vi "Leng Conv.vi"(8 "Unit":bool, 11 "Winding Length":dbl) -> (3 "String":string)   [LabVIEW 2014, in "Programing Logic.lvclass"]
uses:
  Programming Logic/Programing Logic.lvclass
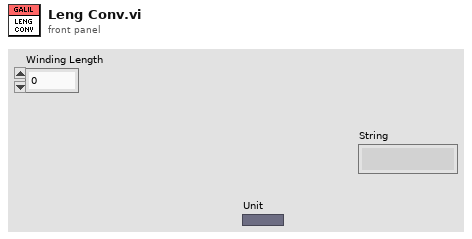
[diagram p1: front panel]
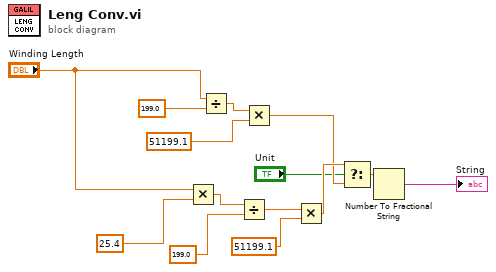
[diagram p0: block diagram]
diagram:
  n1 = Multiply(x="Winding Length", y=25.4) -> (x*y=w6:dbl)
  n2 = Divide(x="Winding Length", y=199.0) -> (x/y=w3:dbl)
  n3 = Divide(x=w6, y=199.0) -> (x/y=w10:dbl)
  n4 = Multiply(x=w3, y=51199.1) -> (x*y=w13:dbl)
  n5 = Multiply(x=w10, y=51199.1) -> (x*y=w14:dbl)
  n6 = Select(t=w14, s="Unit", f=w13) -> (s? t:f=w8:dbl)
  n7 = Number To Fractional String(number=w8) -> (F-format string=→"String":string)  [unwired: 3 in]
